vi "VI Tree.vi"   [LabVIEW 2015, in "Agilent 428X Series.lvlib"]
doc: "This instrument module provides programming support for the HP4284A and 4285A - Precision LCR Meters. They are cost-effective solutions for component and material measurement and can be used to improve component quality by providing an accurate, high throughput test solution. The wide 20Hz to 1MHz (or 75kHz to 30MHz) test frequency range and superior test signal performance allow them to test components to the most commonly used test standards, such as IEC/MIL standards, and under conditions that simulate the intended application.\n\n\nRevised Dated: 11/17/97\nRevised By: DC\nNew Feature Added: Accuracy Calculation, OPEN, SHORT, and\n LOAD Compensation. Interactive execution.\n \nDisclaimer: All accuracy calculation VI's are not part of the original \n driver. They are provided for supplementry purpose only.\n If user desires very high accuracy data, please do or \n check the calculation seperately."
uses:
  <instrlib>/Agilent 428X Series/Agilent 428X Series.lvlib
panel:
  # "© Copyright 2005 National Instruments Corporation.  All Rights Reserved."
  # "SEE DIAGRAM\nFOR VI TREE."
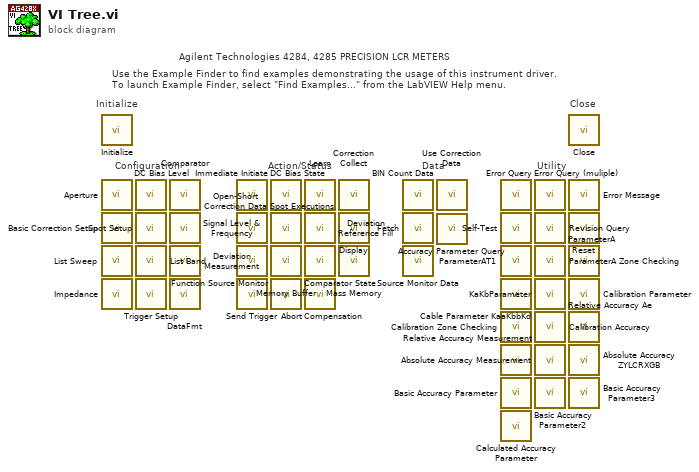
[diagram p0: block diagram]
diagram:
  # "Agilent Technologies 4284, 4285 PRECISION LCR METERS"
  # "Utility"
  # "Data"
  # "Action/Status"
  # "Configuration"
  # "Use the Example Finder to find examples demonstrating the usage of this instrument driver.\nTo launch Example Finder, select \"Find Examples...\" from the LabVIEW Help menu."
  # "Initialize"
  # "Close"
  n1 = call <instrlib>:"Initialize.vi"() -> ()  [unwired: 10 in, 2 out]
  n2 = call <instrlib>:"Aperture.vi"() -> ()  [unwired: 10 in, 2 out]
  n3 = call <instrlib>:"Basic Correction Setup.vi"() -> ()  [unwired: 13 in, 3 out]
  n4 = call <instrlib>:"List Sweep.vi"() -> ()  [unwired: 10 in, 2 out]
  n5 = call <instrlib>:"Impedance.vi"() -> ()  [unwired: 10 in, 2 out]
  n6 = call <instrlib>:"DC Bias Level.vi"() -> ()  [unwired: 10 in, 2 out]
  n7 = call <instrlib>:"Spot Setup.vi"() -> ()  [unwired: 10 in, 2 out]
  n8 = call <instrlib>:"List Band.vi"() -> ()  [unwired: 10 in, 2 out]
  n9 = call <instrlib>:"Trigger Setup.vi"() -> ()  [unwired: 10 in, 2 out]
  n10 = call <instrlib>:"Comparator.vi"() -> ()  [unwired: 18 in, 2 out]
  n11 = call <instrlib>:"Signal Level & Frequency.vi"() -> ()  [unwired: 10 in, 2 out]
  n12 = call <instrlib>:"Deviation Measurement.vi"() -> ()  [unwired: 10 in, 2 out]
  n13 = call <instrlib>:"DataFmt.vi"() -> ()  [unwired: 10 in, 2 out]
  n14 = call <instrlib>:"Immediate Initiate.vi"() -> ()  [unwired: 10 in, 2 out]
  n15 = call <instrlib>:"Open-Short Correction Data.vi"() -> ()  [unwired: 10 in, 2 out]
  n16 = call <instrlib>:"Function Source Monitor.vi"() -> ()  [unwired: 10 in, 2 out]
  n17 = call <instrlib>:"Send Trigger.vi"() -> ()  [unwired: 10 in, 2 out]
  n18 = call <instrlib>:"DC Bias State.vi"() -> ()  [unwired: 10 in, 2 out]
  n19 = call <instrlib>:"Spot Executions.vi"() -> ()  [unwired: 10 in, 2 out]
  n20 = call <instrlib>:"Memory Buffer.vi"() -> ()  [unwired: 10 in, 2 out]
  n21 = call <instrlib>:"Abort.vi"() -> ()  [unwired: 10 in, 2 out]
  n22 = call <instrlib>:"Learn.vi"() -> ()  [unwired: 9 in, 3 out]
  n23 = call <instrlib>:"Deviation Reference Fill.vi"() -> ()  [unwired: 10 in, 2 out]
  n24 = call <instrlib>:"Comparator State.vi"() -> ()  [unwired: 10 in, 2 out]
  n25 = call <instrlib>:"Compensation.VI"() -> ()  [unwired: 14 in, 2 out]
  n26 = call <instrlib>:"Correction Collect.vi"() -> ()  [unwired: 10 in, 2 out]
  n27 = call <instrlib>:"Display.vi"() -> ()  [unwired: 10 in, 2 out]
  n28 = call <instrlib>:"Mass Memory.vi"() -> ()  [unwired: 10 in, 2 out]
  n29 = call <instrlib>:"BIN Count Data.vi"() -> ()  [unwired: 9 in, 3 out]
  n30 = call <instrlib>:"Fetch.vi"() -> ()  [unwired: 9 in, 3 out]
  n31 = call <instrlib>:"Source Monitor Data.vi"() -> ()  [unwired: 8 in, 4 out]
  n32 = call <instrlib>:"Use Correction Data.vi"() -> ()  [unwired: 9 in, 3 out]
  n33 = call <instrlib>:"Accuracy Parameter Query.vi"() -> ()  [unwired: 6 in, 6 out]
  n34 = call <instrlib>:"Error Query.vi"() -> ()  [unwired: 8 in, 4 out]
  n35 = call <instrlib>:"Self-Test.vi"() -> ()  [unwired: 8 in, 4 out]
  n36 = call <instrlib>:"ParameterAT1.vi"() -> ()  [unwired: 9 in, 3 out]
  n37 = call <instrlib>:"Cable Parameter KaaKbbKd.vi"() -> ()  [unwired: 11 in, 5 out]
  n38 = call <instrlib>:"Calibration Zone Checking .vi"() -> ()  [unwired: 9 in, 3 out]
  n39 = call <instrlib>:"Relative Accuracy Measurement.vi"() -> ()  [unwired: 8 in, 8 out]
  n40 = call <instrlib>:"Basic Accuracy Parameter.vi"() -> ()  [unwired: 8 in, 4 out]
  n41 = call <instrlib>:"Calculated Accuracy Parameter.vi"() -> ()  [unwired: 12 in, 4 out]
  n42 = call <instrlib>:"Error Query (muliple).vi"() -> ()  [unwired: 8 in, 4 out]
  n43 = call <instrlib>:"Revision Query.vi"() -> ()  [unwired: 8 in, 4 out]
  n44 = call <instrlib>:"ParameterA Zone Checking.vi"() -> ()  [unwired: 9 in, 3 out]
  n45 = call <instrlib>:"KaKbParameter.vi"() -> ()  [unwired: 8 in, 4 out]
  n46 = call <instrlib>:"Calibration Accuracy.vi"() -> ()  [unwired: 8 in, 4 out]
  n47 = call <instrlib>:"Absolute Accuracy Measurement.vi"() -> ()  [unwired: 12 in, 8 out]
  n48 = call <instrlib>:"Basic Accuracy Parameter2.vi"() -> ()  [unwired: 8 in, 8 out]
  n49 = call <instrlib>:"Close.vi"() -> ()  [unwired: 11 in, 1 out]
  n50 = call <instrlib>:"Error Message.vi"() -> ()  [unwired: 7 in, 5 out]
  n51 = call <instrlib>:"Reset.vi"() -> ()  [unwired: 10 in, 2 out]
  n52 = call <instrlib>:"ParameterA.vi"() -> ()  [unwired: 13 in, 3 out]
  n53 = call <instrlib>:"Calibration Parameter.vi"() -> ()  [unwired: 9 in, 3 out]
  n54 = call <instrlib>:"Relative Accuracy Ae.vi"() -> ()  [unwired: 17 in, 3 out]
  n55 = call <instrlib>:"Absolute Accuracy ZYLCRXGB.vi"() -> ()  [unwired: 9 in, 3 out]
  n56 = call <instrlib>:"Basic Accuracy Parameter3.vi"() -> ()  [unwired: 8 in, 4 out]
